vi "Get Times.vi"(8 "error in (no error)":errorcluster, 9 "End Time":timestamp, 10 "Start Time":timestamp, 11 "User Interface in":refnum<class "User Interface.lvclass">) -> (0 "error out":errorcluster, 3 "User Interface out":refnum<class "User Interface.lvclass">)   [LabVIEW 2020, in "User Interface.lvlib" / "User Interface.lvclass"]
uses:
  User Interface.lvclass
  User Interface.lvclass/User Interface.ctl
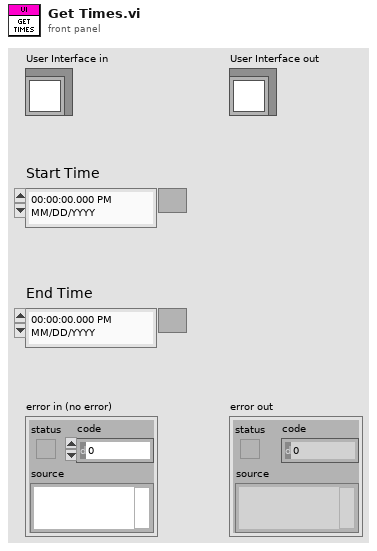
[diagram p1: front panel]
types:
  T1 = typedef "LVDateTimeRec.ctl" = cluster{"fractional second":dbl, "second":i32, "minute":i32, "hour":i32, "day of month":i32, "month":i32, "year":i32, "day of week":i32, "day of year":i32, "DST":i32}
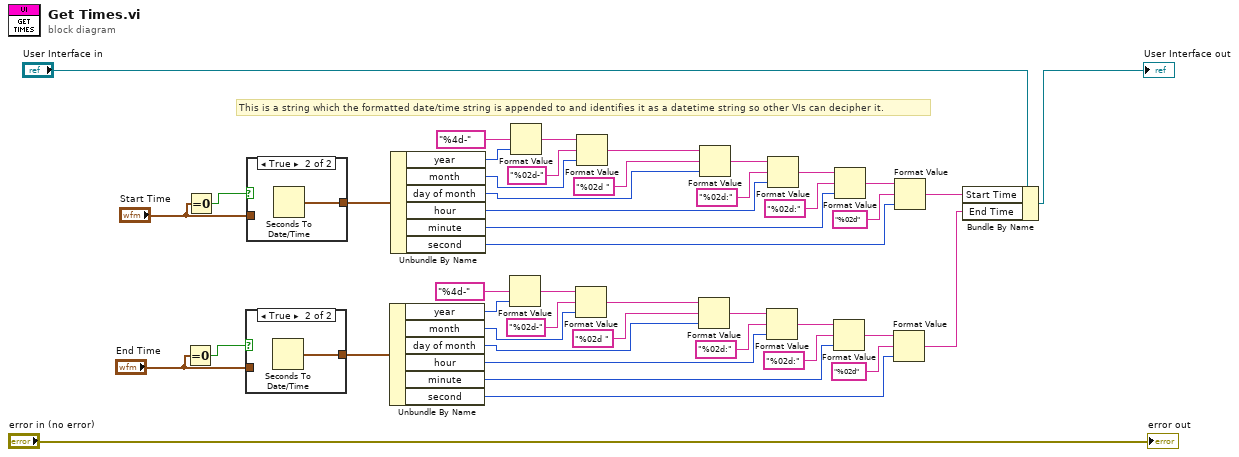
[diagram p0: block diagram]
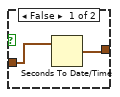
[diagram p2: hidden frame]
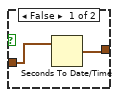
[diagram p3: hidden frame]
diagram:
  # "This is a string which the formatted date/time string is appended to and identifies it as a datetime string so other VIs can decipher it."
  n1 = Equal To 0?(x="End Time") -> (x = 0?=w3:bool)
  n2 = Equal To 0?(x="Start Time") -> (x = 0?=w41:bool)
  n3 = case shown="True" w3 {
    tunnel: [w46 w48] -> w4
    tunnel: "End Time" -> [w47 _]
    frame False {
      n4 = Seconds To Date/Time(time stamp (now)=w47) -> (date time rec=w46:T1)  [unwired: 1 in]
    }
    frame True {
      n5 = Seconds To Date/Time() -> (date time rec=w48:T1)  [unwired: 2 in]
    }
  }
  n6 = case shown="True" w41 {
    tunnel: [w49 w51] -> w40
    tunnel: "Start Time" -> [w50 _]
    frame False {
      n7 = Seconds To Date/Time(time stamp (now)=w50) -> (date time rec=w49:T1)  [unwired: 1 in]
    }
    frame True {
      n8 = Seconds To Date/Time() -> (date time rec=w51:T1)  [unwired: 2 in]
    }
  }
  n9 = Unbundle By Name(w4) -> ("year"=w9:i32, "month"=w8:i32, "day of month"=w7:i32, "hour"=w21:i32, "minute"=w18:i32, "second"=w17:i32)
  n10 = Unbundle By Name(w40) -> ("year"=w35:i32, "month"=w36:i32, "day of month"=w37:i32, "hour"=w23:i32, "minute"=w26:i32, "second"=w27:i32)
  n11 = Format Value(format string="%4d-", value (0)=w9) -> (output string=w12:string)  [unwired: 1 in]
  n12 = Format Value(format string="%4d-", value (0)=w35) -> (output string=w32:string)  [unwired: 1 in]
  n13 = Format Value(string ("")=w12, format string="%02d-", value (0)=w8) -> (output string=w11:string)
  n14 = Format Value(string ("")=w32, format string="%02d-", value (0)=w36) -> (output string=w33:string)
  n15 = Format Value(string ("")=w11, format string="%02d ", value (0)=w7) -> (output string=w10:string)
  n16 = Format Value(string ("")=w33, format string="%02d ", value (0)=w37) -> (output string=w34:string)
  n17 = Format Value(string ("")=w10, format string="%02d:", value (0)=w21) -> (output string=w20:string)
  n18 = Format Value(string ("")=w34, format string="%02d:", value (0)=w23) -> (output string=w24:string)
  n19 = Format Value(string ("")=w20, format string="%02d:", value (0)=w18) -> (output string=w19:string)
  n20 = Format Value(string ("")=w24, format string="%02d:", value (0)=w26) -> (output string=w25:string)
  n21 = Format Value(string ("")=w19, format string="%02d", value (0)=w17) -> (output string=w1:string)
  n22 = Format Value(string ("")=w25, format string="%02d", value (0)=w27) -> (output string=w22:string)
  n23 = Bundle By Name(cluster="User Interface in", "Start Time"=w22, "End Time"=w1) -> (→"User Interface out":refnum<class "User Interface.lvclass">)
  "error out" <- "error in (no error)"
